vi "calculateFromSubset.vi"(0 "CRC16 in":refnum<class "CRC16.lvclass">, 5 "Data":u8[](array[numeric]), 7 "StartIndex":i32, 9 "Length":i32, 11 "error in (no error)":errorcluster) -> (4 "CRC16 out":refnum<class "CRC16.lvclass">, 6 "CRC":u16 format="%0d", 15 "error out":errorcluster)   [LabVIEW 2016, in "RTUtilities.lvlib" / "CRC16.lvclass"]
uses:
  CRC16.lvclass
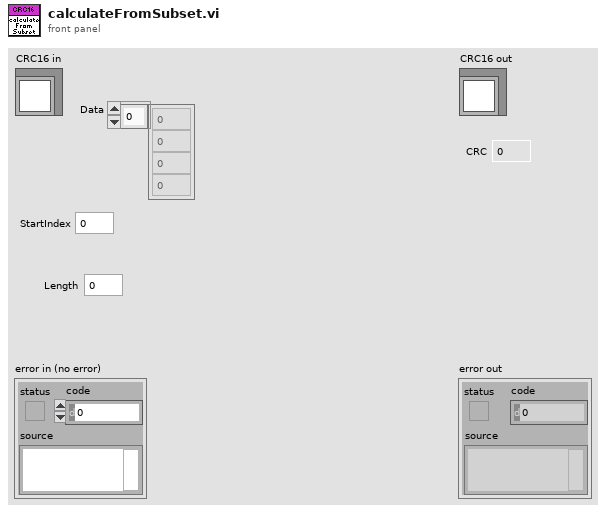
[diagram p1: front panel]
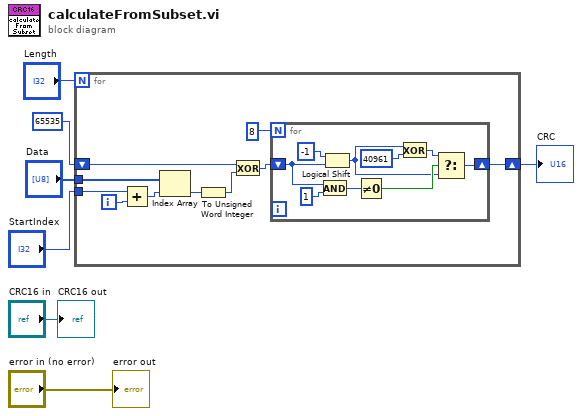
[diagram p0: block diagram]
diagram:
  n1 = for {
    N: "Length" -> [_]
    tunnel: "Data" -> [w12]
    shift-right: [w14] -> w6
    shift-left: u16 65535 -> [w16]
    tunnel: "StartIndex" -> [w10]
    i -> [w11]
    n2 = Add(x=w10, y=w11) -> (x+y=w9:i32)
    n3 = Index Array(array=w12, index=w9) -> (element=w8:u8)
    n4 = To Unsigned Word Integer(number=w8) -> (unsigned 16bit integer=w13:u16)
    n5 = Exclusive Or(1:w13, 2:w16) -> (0:w15:u16)
    n6 = for {
      N: 8 -> [_]
      shift-right: [w19] -> w14
      shift-left: w15 -> [w20]
      n7 = And(x=w20, y=u16 1) -> (x .and. y?=w26:u16)
      n8 = Logical Shift(y=i16 -1, x=w20) -> (x << y=w18:u16)
      n9 = Not Equal To 0?(x=w26) -> (x != 0?=w25:bool)
      n10 = Exclusive Or(1:u16 40961 ("y"), 2:w18) -> (0:w21:u16)
      n11 = Select(t=w21, s=w25, f=w18) -> (s? t:f=w19:u16)
    }
  }
  "CRC" <- w6
  "error out" <- "error in (no error)"
  "CRC16 out" <- "CRC16 in"
